vi "Get Latest Data.vi"(7 "LabVIEW Web Service Request":refnum<class "Web Request.lvclass">) -> (0 "Temperature":dbl, 1 "Wind Speed":dbl, 2 "Wind Direction":dbl, 3 "Pressure":dbl)   [LabVIEW 2023]
doc: "HTTP method VI that retrieves the latest weather data and outputs it using terminal-mode output."
uses:
  <vilib>/wsapi/Web Request.lvclass
  Application/Weather Data.lvlib
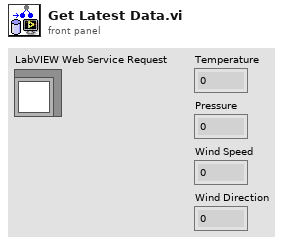
[diagram p1: front panel]
types:
  T1 = typedef "Weather Data.lvlib/Weather Data.ctl" = cluster{"Temperature":dbl, "Pressure":dbl, "Wind Speed":dbl, "Wind Direction":dbl}
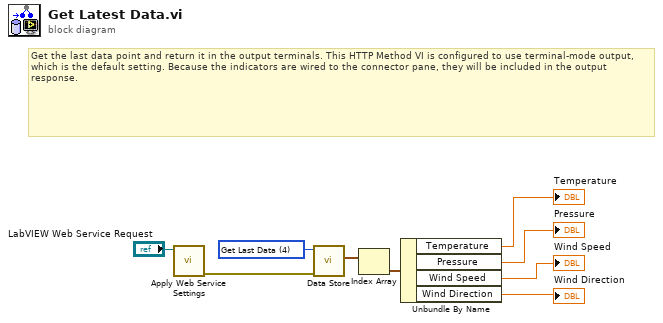
[diagram p0: block diagram]
diagram:
  w9 = u16 4 items=["Initialize Data Store", "Destroy Data Store", "Clear Data", "Append Data", "Get Last Data", "Get All Data"] ("action")
  # "Get the last data point and return it in the output terminals. This HTTP Method VI is configured to use terminal-mode output, which is the default setting. Because the indicators are wired to the connector pane, they will be included in the output response."
  n1 = call "Apply Web Service Settings.vi"("LabVIEW Web Service Request"="LabVIEW Web Service Request") -> ("error out"=w2:errorcluster)  [unwired: 9 in, 1 out]
  n2 = call "Data Store.vi"("error in (no error)"=w2, "action"=w9) -> ("weather data out"=w8:T1[])  [unwired: 8 in, 1 out]
  n3 = Index Array(array=w8) -> (element=w7:T1)  [unwired: 1 in]
  n4 = Unbundle By Name(w7) -> ("Temperature"=→"Temperature":dbl, "Pressure"=→"Pressure":dbl, "Wind Speed"=→"Wind Speed":dbl, "Wind Direction"=→"Wind Direction":dbl)
